vi "execution class name.vi"(8 "error in":errorcluster, 11 "current tag file io module configuration in":refnum<class "file io module configuration.lvclass">) -> (0 "error out":errorcluster, 2 "class name":string, 3 "current tag file io module configuration out":refnum<class "file io module configuration.lvclass">)   [LabVIEW 2013, in "file io module configuration.lvclass"]
doc: "Provides an interface for determining the module runtime class associated with this module configuration. This class name can then be used to dynamically load or locate the runtime class for initialization purposes."
uses:
  file io module configuration.lvclass
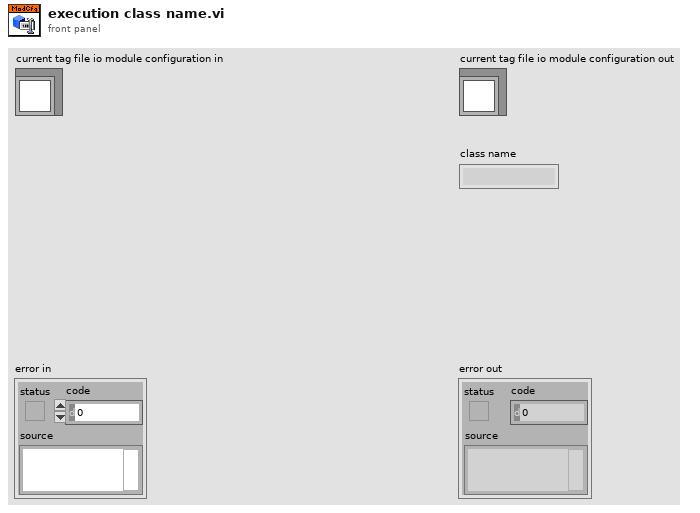
[diagram p1: front panel]
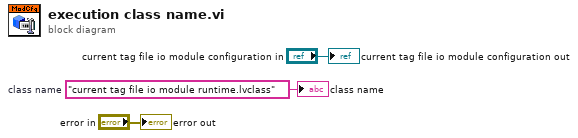
[diagram p0: block diagram]
diagram:
  w1 = "current tag file io module runtime.lvclass"  # class name
  "error out" <- "error in"
  "current tag file io module configuration out" <- "current tag file io module configuration in"
  "class name" <- w1
